vi "CH_LM Self-Test.vi"(0 "Meter Index":i32, 5 "error in (no error)":errorcluster, 7 "Timeout / ms (3000)":i32=3000, 9 "Lock Timeout / ms (1000)":i32=1000) -> (11 "Lock timed out":bool, 14 "Meter Index":i32, 15 "Self-Test Result Code":i32, 18 "Self-Test Result Message":string, 19 "error out":errorcluster)   [LabVIEW 2012, in "CH_LM.lvlib"]
doc: "Runs the instrument's self-test routine and returns the test results."
uses:
  CH_LM.lvlib
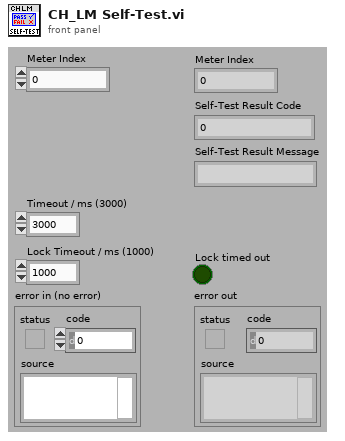
[diagram p1: front panel]
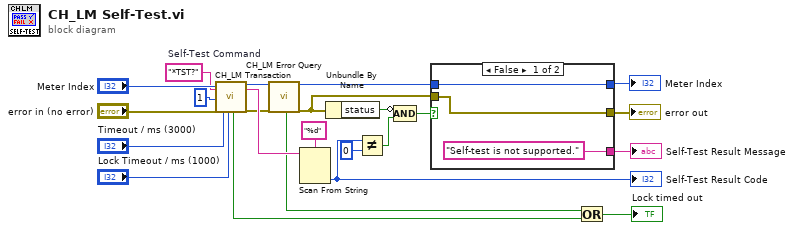
[diagram p0: block diagram]
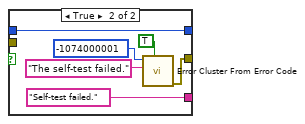
[diagram p2: hidden frame]
diagram:
  w14 = "*TST?"  # Self-Test Command
  n1 = call "CH_LM Transaction.vi"("Meter Index"="Meter Index", "Command String"=w14, "NofStrings (-1:all)"=1, "error in (no error)"="error in (no error)", "Timeout / ms (3000)"="Timeout / ms (3000)", "Lock Timeout / ms (1000)"="Lock Timeout / ms (1000)") -> ("Lock timed out"=w4:bool, "Meter Index"=w8:i32, "Response"=w16:string, "error out"=w6:errorcluster)  [unwired: 10 out]
  n2 = call "CH_LM Error Query.vi"("Meter Index"=w8, "error in (no error)"=w6) -> ("Lock timed out"=w2:bool, "Meter Index"=w7:i32, "error out"=w5:errorcluster)  [unwired: 15 out]
  n3 = Scan From String(format string="%d", input string=w16) -> (output 1=w19:i32)  [unwired: 2 in, 4 out]
  "Self-Test Result Code" <- w19
  n4 = Unbundle By Name(w5) -> ("status"=w21:bool)
  n5 = Not Equal?(x=w19, y=0) -> (x != y?=w22:bool)
  n6 = Compound Arithmetic op=AND(invert w21, w22) -> (w20:bool)
  n7 = case shown="False" w20 {
    tunnel: w7 -> [w26 w32]
    tunnel: w5 -> [w25 _]
    tunnel: [w25 w28] -> w12
    tunnel: [w26 w32] -> w13
    tunnel: ["Self-test is not supported." ("Source (VI Name)") "Self-test failed." ("Source (VI Name)")] -> w1
    frame False {
    }
    frame True {
      n8 = call <vilib>:"Error Cluster From Error Code.vi"("show call chain? (False)"=TRUE, "error message (\"\")"="The self-test failed." ("Source (VI Name)"), "error code (0)"=-1074000001 ("Code")) -> ("error out"=w28:errorcluster)  [unwired: 1 in, 5 out]
    }
  }
  "Self-Test Result Message" <- w1
  "Meter Index" <- w13
  "error out" <- w12
  n9 = Or(x=w2, y=w4) -> (x .or. y?=→"Lock timed out":bool)
